vi "Write Boolean.vi"(8 "error in (no error)":errorcluster, 10 "Boolean":bool, 11 "Basic Class in":refnum<class "Basic Class.lvclass">) -> (0 "error out":errorcluster, 3 "Basic Class out":refnum<class "Basic Class.lvclass">)   [LabVIEW 2020, in "Basic Class.lvclass"]
uses:
  Basic Class.lvclass
  Basic Class.lvclass/Basic Class.ctl
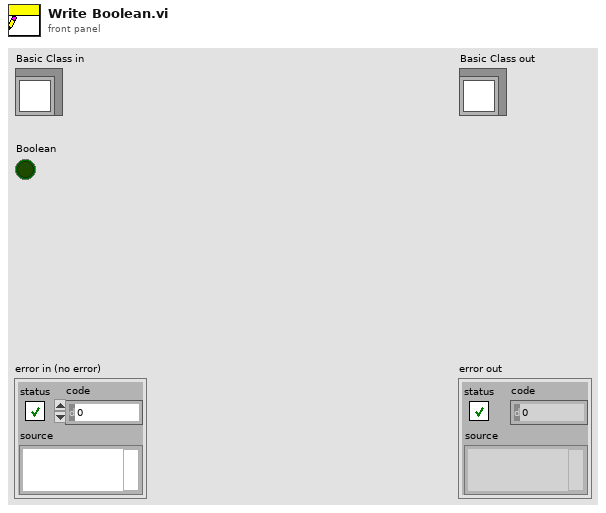
[diagram p1: front panel]
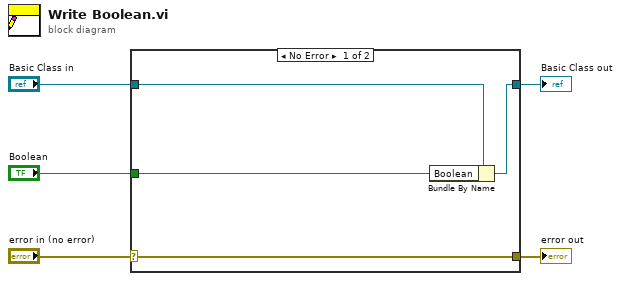
[diagram p0: block diagram]
diagram:
  n1 = case shown="No Error" "error in (no error)" {
    selector: "error in (no error)" -> [w9 w10]
    tunnel: [w9 w10] -> w4
    tunnel: [w7 w11] -> w2
    tunnel: "Basic Class in" -> [w8 w11]
    tunnel: "Boolean" -> [w6 _]
    frame No Error {
      n2 = Bundle By Name(cluster=w8, "Boolean"=w6) -> (w7:refnum<class "Basic Class.lvclass">)
    }
    frame Error {
    }
  }
  "error out" <- w4
  "Basic Class out" <- w2
